vi "msg_handler.vi"(10 "latest notification":T1) -> ()   [LabVIEW 2013]
uses:
  status.ctl
panel:
  # "Status"
  # "Use this to, e.g. update a MySQL log."
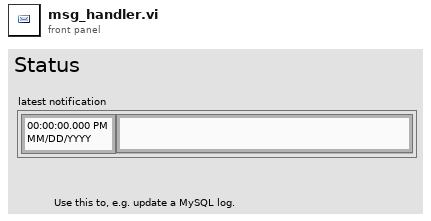
[diagram p1: front panel]
types:
  T1 = typedef "status.ctl" = cluster{"seconds since 1Jan1904":timestamp, string}
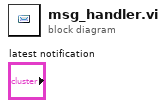
[diagram p0: block diagram]
diagram:
